vi "Publish DO.vi"(8 "error in":errorcluster, 10 "DO Data":bool[](array[boolean]), 11 "BNT_DAQmx-MCSV in":refnum<class "BNT_DAQmx-MCSV.lvclass">) -> (0 "error out":errorcluster, 3 "BNT_DAQmx-MCSV out":refnum<class "BNT_DAQmx-MCSV.lvclass">)   [LabVIEW 2017, in "BNT_DAQmx.lvlib" / "BNT_DAQmx-MCSV.lvclass"]
doc: "Publish digital output values if changed."
uses:
  BNT_DAQmx-MCSV.lvclass
  BNT_DAQmx-MCSV.lvclass/BNT_DAQmx-MCSV.ctl
  CSPP_Core/Classes/CSPP_ProcessVariables/PVConnection/PVConnection.lvclass/PVConnection.ctl
  CSPP_Core/Classes/CSPP_ProcessVariables/ProcessVariable/PV.lvclass/PV.ctl
  CSPP_Core/Classes/CSPP_ProcessVariables/ProcessVariable/Write Data.vi
  CSPP_Core/Classes/CSPP_ProcessVariables/ProcessVariable/Write Error.vi
  CSPP_Core/Classes/CSPP_ProcessVariables/ProcessVariable/Write Quality.vi
  CSPP_Core/Classes/CSPP_ProcessVariables/ProcessVariable/Write status.vi
  CSPP_Core/Classes/CSPP_ProcessVariables/ProcessVariable/Write Timestamp.vi
  CSPP_Core/Classes/CSPP_ProcessVariables/ProcessVariable/PV.lvclass
  CSPP_Core/Classes/CSPP_ProcessVariables/PVConnection/PVConnection.lvclass
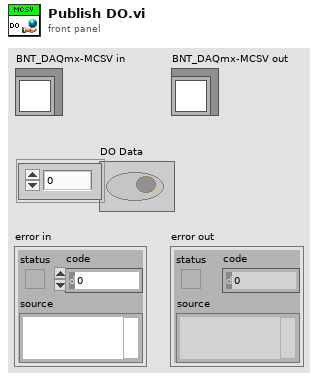
[diagram p1: front panel]
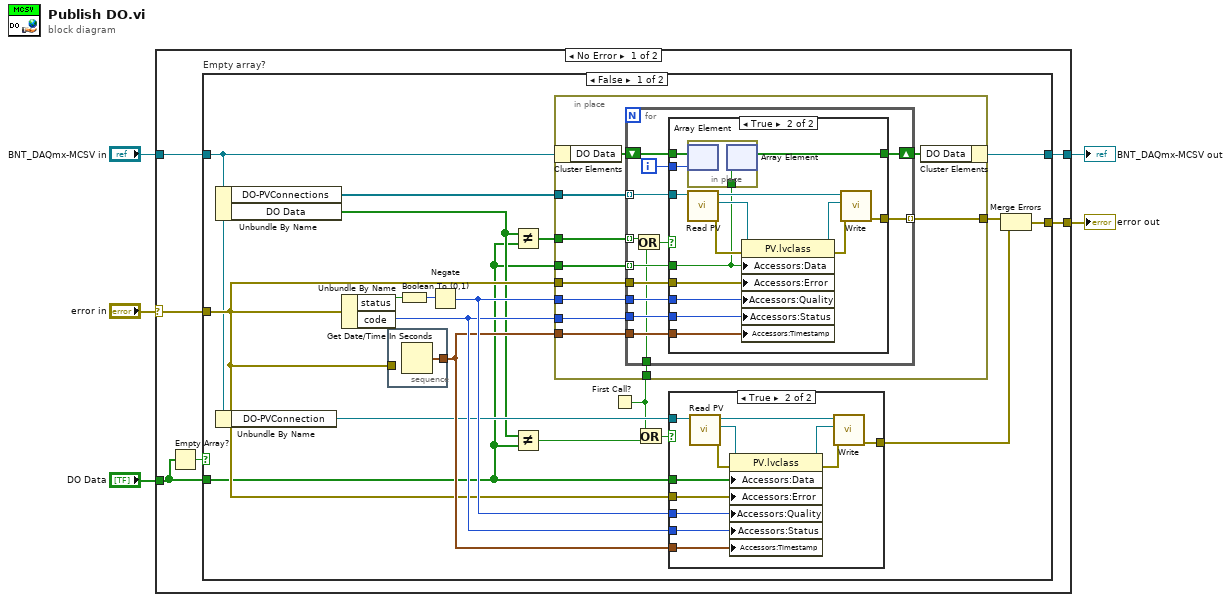
[diagram p0: block diagram]
diagram:
  n1 = case shown="No Error" "error in" {
    selector: "error in" -> [w11 w90]
    tunnel: [w10 w90] -> w4
    tunnel: [w8 w89] -> w2
    tunnel: "BNT_DAQmx-MCSV in" -> [w9 w89]
    tunnel: "DO Data" -> [w6 _]
    frame No Error {
      n2 = Empty Array?(array=w6) -> (empty?=w7:bool)
      n3 = case "Empty array?" shown="False" w7 {
        tunnel: w11 -> [w23 w87]
        tunnel: [w21 w87] -> w10
        tunnel: w9 -> [w16 w88]
        tunnel: [w15 w88] -> w8
        tunnel: w6 -> [w13 _]
        frame False {
          n4 = Unbundle By Name(w16) -> ("DO-PVConnections"=w22:refnum<class "PVConnection.lvclass">[], "DO Data"=w18:bool[])
          n5 = Unbundle By Name(w16) -> ("DO-PVConnection"=w20:refnum<class "PVConnection.lvclass">)
          n6 = Unbundle By Name(w23) -> ("status"=w29:bool, "code"=w26:i32)
          n7 = stacked-sequence {
            tunnel: [w31] -> w25
            tunnel: w23 -> [_]
            frame #0 {
              n8 = Get Date/Time In Seconds() -> (seconds since 1Jan1904=w31:timestamp)
            }
          }
          n9 = Boolean To (0,1)(Boolean=w29) -> (0, 1=w28:i16)
          n10 = Negate(x=w28) -> (-x=w27:i16)
          n11 = Not Equal?(x=w18, y=w13) -> (x != y?=w19:bool[])
          n12 = Not Equal?(x=w18, y=w13) -> (x != y?=w17:bool)
          n13 = First Call?() -> (First Call?: T/F=w12:bool)
          n14 = in-place {
            in-place-border: [w42] -> w30
            in-place-border: w27 -> [w41]
            in-place-border: w26 -> [w40]
            in-place-border: w25 -> [w39]
            in-place-border: w23 -> [w38]
            in-place-border: w22 -> [w37]
            in-place-border: w13 -> [w36]
            in-place-border: w19 -> [w35]
            in-place-border: w12 -> [w32]
            n15 = in-place-cluster #1(w16) -> ("DO Data"=w34:bool[])
            n16 = for {
              tunnel: w37 -> [w49] mode=indexing
              tunnel: w36 -> [w55] mode=indexing
              tunnel: w38 -> [w54]
              tunnel: [w53] -> w42 mode=indexing
              tunnel: w41 -> [w52]
              tunnel: w40 -> [w51]
              tunnel: w39 -> [w50]
              tunnel: w35 -> [w48] mode=indexing
              shift-right: [w45] -> w33
              shift-left: w34 -> [w46]
              tunnel: w32 -> [w43]
              i -> [w47]
              n17 = Or(x=w48, y=w43) -> (x .or. y?=w44:bool)
              n18 = case shown="True" w44 {
                tunnel: w55 -> [_ w59]
                tunnel: w54 -> [w57 w72]
                tunnel: [w57 w69] -> w53
                tunnel: w52 -> [_ w68]
                tunnel: w51 -> [_ w67]
                tunnel: w50 -> [_ w66]
                tunnel: w49 -> [_ w65]
                tunnel: w47 -> [_ w61]
                tunnel: w46 -> [w56 w60]
                tunnel: [w56 w58] -> w45
                frame False {
                }
                frame True {
                  n19 = in-place {
                    in-place-border: w59 -> [w73]
                    n20 = in-place-array #2(w60, w61) -> ()  [unwired: 1 out]
                    n21 = in-place-array #2(w73) -> (w58:bool[])  [unwired: 1 out]
                  }
                  n22 = call "Read PV.vi"("PVConnection in"=w65) -> ("error out"=w62:errorcluster, "PV"=w63:refnum<class "PV.lvclass">, "PVConnection out"=w64:refnum<class "PVConnection.lvclass">)  [unwired: 8 in]
                  n23 = property class="PV.lvclass"(reference=w63, error in=w62, "Accessors:Data"=w59, "Accessors:Error"=w72, "Accessors:Quality"=w68, "Accessors:Status"=w67, "Accessors:Timestamp"=w66) -> (reference out=w71:refnum<class "PV.lvclass">, error out=w70:errorcluster)
                  n24 = call "Write.vi"("error in (no error)"=w70, "PV"=w71, "PVConnection in"=w64) -> ("error out"=w69:errorcluster)  [unwired: 7 in, 1 out]
                }
              }
            }
            n25 = in-place-cluster #1("DO Data"=w33) -> (w15:refnum<class "BNT_DAQmx-MCSV.lvclass">)
          }
          n26 = Or(x=w12, y=w17) -> (x .or. y?=w14:bool)
          n27 = case shown="True" w14 {
            tunnel: w27 -> [_ w81]
            tunnel: w26 -> [_ w80]
            tunnel: w25 -> [_ w79]
            tunnel: [w74 w78] -> w24
            tunnel: w23 -> [w74 w77]
            tunnel: w20 -> [_ w76]
            tunnel: w13 -> [_ w75]
            frame False {
            }
            frame True {
              n28 = call "Read PV.vi"("PVConnection in"=w76) -> ("error out"=w82:errorcluster, "PV"=w83:refnum<class "PV.lvclass">, "PVConnection out"=w84:refnum<class "PVConnection.lvclass">)  [unwired: 8 in]
              n29 = property class="PV.lvclass"(reference=w83, error in=w82, "Accessors:Data"=w75, "Accessors:Error"=w77, "Accessors:Quality"=w81, "Accessors:Status"=w80, "Accessors:Timestamp"=w79) -> (reference out=w86:refnum<class "PV.lvclass">, error out=w85:errorcluster)
              n30 = call "Write.vi"("error in (no error)"=w85, "PV"=w86, "PVConnection in"=w84) -> ("error out"=w78:errorcluster)  [unwired: 7 in, 1 out]
            }
          }
          n31 = Merge Errors(w30, w24) -> (w21:errorcluster)
        }
        frame True {
        }
      }
    }
    frame Error {
    }
  }
  "error out" <- w4
  "BNT_DAQmx-MCSV out" <- w2
